vi "interruptible_wait.vi"(9 "profile_time":u32, 11 "Fehler (Eingang)":errorcluster) -> (3 "Fehler (Ausgang)":errorcluster)   [LabVIEW 2013]
uses:
  global_notaus.vi
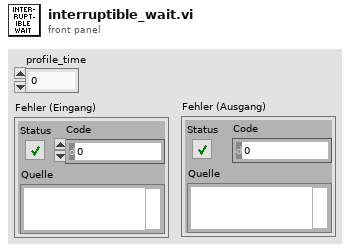
[diagram p1: front panel]
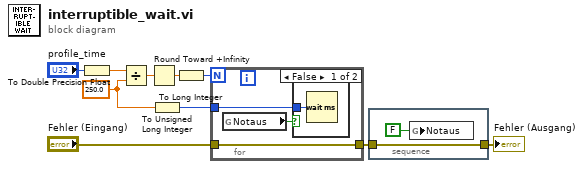
[diagram p0: block diagram]
diagram:
  w5 = 250.0 ("y")
  n1 = To Double Precision Float(number="profile_time") -> (double precision float=w9:dbl)
  n2 = Divide(x=w9, y=w5) -> (x/y=w8:dbl)
  n3 = Round Toward +Infinity(x=w8) -> (ceil(x): smallest int >= x=w7:dbl)
  n4 = To Unsigned Long Integer(number=w5) -> (unsigned 32bit integer=w4:u32)
  n5 = To Long Integer(number=w7) -> (32bit integer=w6:i32)
  n6 = for {
    N: w6 -> [_]
    tunnel: w4 -> [w13]
    tunnel: [w11] -> w2
    tunnel: "Fehler (Eingang)" -> [w11]
    n7 = global read "global_notaus.vi" "Notaus"() -> (w12:bool)
    n8 = case shown="False" w12 {
      tunnel: w13 -> [w14 _]
      frame False {
        n9 = Wait (ms)(milliseconds to wait=w14) -> ()  [unwired: 1 out]
      }
      frame True {
      }
    }
  }
  n10 = stacked-sequence {
    tunnel: w2 -> [w16]
    tunnel: [w16] -> w1
    frame #0 {
      n11 = global write "global_notaus.vi" "Notaus"(FALSE) -> ()
    }
  }
  "Fehler (Ausgang)" <- w1
